vi "SimpleConsoleExample.vi"() -> ()   [LabVIEW 2016]
doc: "This example VI implements an interactive console for sending/retrieving commands and data to and from Hyperion instruments."
uses:
  h.Library/COMM/CTL/h.COMM.Command Status Enum.ctl
  <vilib>/Utility/miscctls.llb/LVPointTypeDef.ctl
  <vilib>/Utility/miscctls.llb/LVRectTypeDef.ctl
  h.Library/COMM/CTL/h.COMM.Socket Type.ctl
  h.Library.lvlib
panel:
  in  "Stop Button":bool
  in  "ip address:":string="10.0.0.55"
  in  "Execute":bool
  out "Content":u8[](array[numeric])
  out "Status":T1
  out "Message":string
  in  "Command":string
  # "hyperion simple console example"
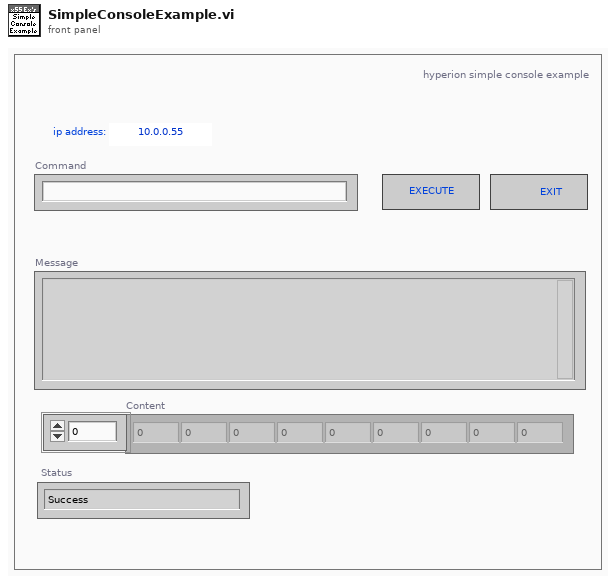
[diagram p1: front panel]
types:
  T1 = typedef "h.Library.lvlib/h.COMM.Command Status Enum.ctl" = enum8{"Success", "Failed", "Error", "AccessDenied", "InvalidCommand", "InvalidNumberArguments", "InvalidArgument", ""}
  T2 = typedef "LVRectTypeDef.ctl" = cluster{"Left":i16, "Top":i16, "Right":i16, "Bottom":i16}
  T3 = typedef "LVPointTypeDef.ctl" = cluster{"Horizontal":i16, "Vertical":i16}
  T4 = typedef "h.Library.lvlib/h.COMM.Socket Type.ctl" = u16
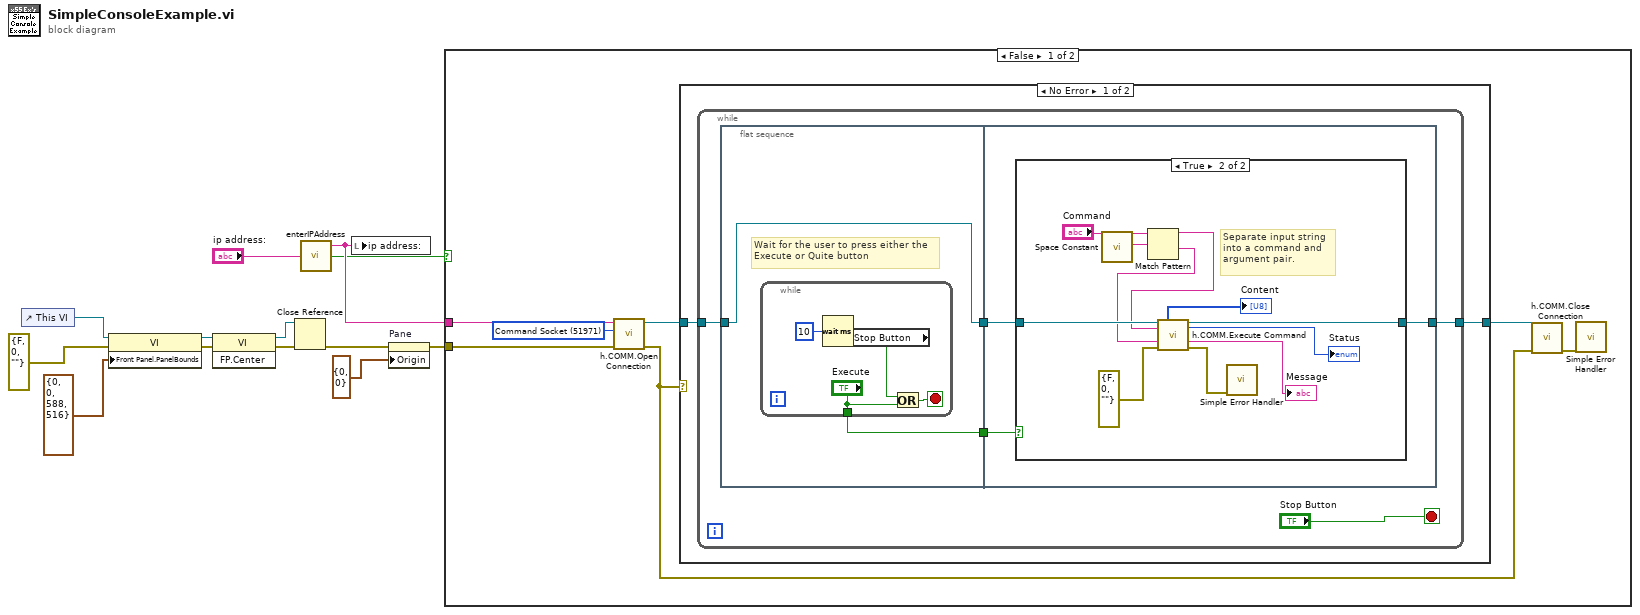
[diagram p0: block diagram]
diagram:
  n1 = control-ref of="This VI"() -> (w13:refnum<vi>)
  n2 = property class="VI"(reference=w13, error in=errorcluster {"status"=FALSE, "code"=0, "source"=""}, "Front Panel.PanelBounds"=T2 {"Left"=0, "Top"=0, "Right"=588, "Bottom"=516} ("Front Panel Window:Panel Bounds 2")) -> (reference out=w12:refnum<vi>, error out=w10:errorcluster)
  n3 = invoke class="VI" method="FP.Center"(reference=w12, error in=w10) -> (reference out=w8:refnum<vi>, error out=w7:errorcluster)  [unwired: 1 in, 1 out]
  n4 = Close Reference(reference=w8, error in (no error)=w7) -> (error out=w6:errorcluster)
  n5 = call "enterIPAddress.vi"("IP Address"="ip address:") -> ("IP Address Out"=w2:string, "Was Canceled"=w1:bool)  [unwired: 1 in]
  n6 = local write "ip address:"(w2) -> ()
  n7 = property on="Pane" class="Pane"(error in=w6, "Origin"=T3 {"Horizontal"=0, "Vertical"=0}) -> (error out=w4:errorcluster)  [unwired: 1 in, 1 out]
  n8 = case shown="False" w1 {
    tunnel: w4 -> [w15 _]
    tunnel: w2 -> [w14 _]
    frame False {
      w16 = T4 51971 items=["Command Socket"=51971, "Streaming Data Socket"=51972] ("Port")
      n9 = call "h.COMM.Open Connection.vi"("error in"=w15, "Port"=w16, "Address"=w14) -> ("error out"=w18:errorcluster, "Connection ID"=w20:refnum<k5>)  [unwired: 7 in]
      n10 = case shown="No Error" w18 {
        tunnel: w20 -> [w22 w49]
        tunnel: [w21 w49] -> w19
        frame No Error {
          n11 = while {
            tunnel: w22 -> [w25]
            tunnel: [w24] -> w21
            stop <- "Stop Button" stop-if-true
            n12 = flat-sequence {
              tunnel: w25 -> [w29]
              tunnel: [w29] -> w27
              tunnel: [w28] -> w26
              tunnel: [w35] -> w24
              tunnel: w27 -> [w36]
              tunnel: w26 -> [w34]
              frame #0 {
                # "Wait for the user to press either the\nExecute or Quite button"
                n13 = while {
                  tunnel: ["Execute"] -> w28
                  stop <- w32 stop-if-true
                  n14 = Wait (ms)(milliseconds to wait=u32 10) -> ()  [unwired: 1 out]
                  n15 = local read "Stop Button"() -> (w31:bool)
                  n16 = Or(x=w31, y="Execute") -> (x .or. y?=w32:bool)
                }
              }
              frame #1 {
                n17 = case shown="True" w34 {
                  tunnel: w36 -> [w37 w48]
                  tunnel: [w37 w47] -> w35
                  frame False {
                  }
                  frame True {
                    # "Separate input string\ninto a command and\nargument pair."
                    n18 = call <vilib>:"Space Constant.vi"() -> ("String"=w42:string)
                    n19 = Match Pattern(string="Command", regular expression=w42) -> (before substring=w40:string, after substring=w39:string)  [unwired: 1 in, 2 out]
                    n20 = call "h.COMM.Execute Command.vi"("Connection ID"=w48, "Command"=w40, "Argument"=w39, "error in"=errorcluster {"status"=FALSE, "code"=0, "source"=""}) -> ("Content"=→"Content":u8[], "Status"=→"Status":T1, "Connection ID out"=w47:refnum<k5>, "Message"=→"Message":string, "error out"=w44:errorcluster)  [unwired: 4 in, 3 out]
                    n21 = call <vilib>:"Simple Error Handler.vi"("error in (no error)"=w44) -> ()  [unwired: 4 in, 5 out]
                  }
                }
              }
            }
          }
        }
        frame Error {
        }
      }
      n22 = call "h.COMM.Close Connection.vi"("error in"=w18, "Connection ID"=w19) -> ("error out"=w17:errorcluster)  [unwired: 9 in]
      n23 = call <vilib>:"Simple Error Handler.vi"("error in (no error)"=w17) -> ()  [unwired: 4 in, 5 out]
    }
    frame True {
    }
  }
